vi "REACTOR_PARSE_SET_TEMPERATURAS.vi"(11 "String":string="CALOR : 25.0C a  25.0C/min, FRIO: 20.0C a  25.0C/min, y espera a estabilizar") -> (0 "RAMPA_F (C/MIN)":dbl=25.0, 1 "FRIO (C)":dbl=20.0, 2 "RAMPA_C (C/MIN)":dbl=25.0, 3 "CALOR (C)":dbl=25.0, 5 "T.Wait Stability":bool)   [LabVIEW 2017]
panel:
  out "subString":string
  # "CALOR : 25.0C a  25.0C/min, FRIO: 20.0C a  25.0C/min, y espera a estabilizar"
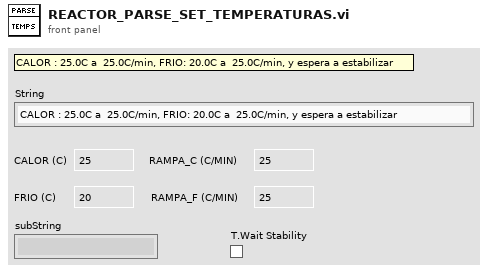
[diagram p1: front panel]
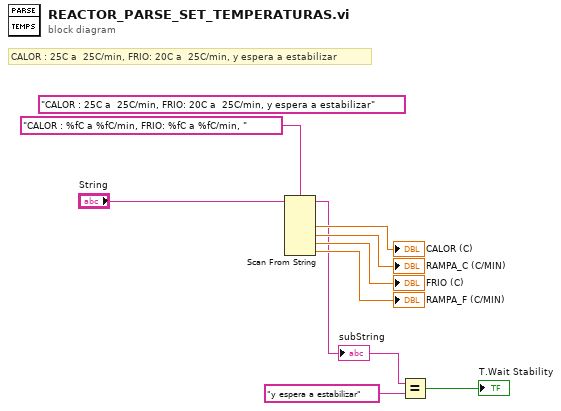
[diagram p0: block diagram]
diagram:
  (unwired) "CALOR : 25C a  25C/min, FRIO: 20C a  25C/min, y espera a estabilizar" ("format string")
  # "CALOR : 25C a  25C/min, FRIO: 20C a  25C/min, y espera a estabilizar"
  n1 = Scan From String(format string="CALOR : %fC a %fC/min, FRIO: %fC a %fC/min, ", input string="String") -> (remaining string=w1:string, output 1=→"CALOR (C)":dbl, output 2=→"RAMPA_C (C/MIN)":dbl, output 3=→"FRIO (C)":dbl, output 4=→"RAMPA_F (C/MIN)":dbl)  [unwired: 6 in, 2 out]
  "subString" <- w1
  n2 = Equal?(x=w1, y="y espera a estabilizar" ("after substring")) -> (x = y?=→"T.Wait Stability":bool)
